vi "Update.vi"(8 "error in (no error)":errorcluster, 10 "Message in":refnum<class "UpdateMessage.lvclass">, 11 "Retiga in":refnum<class "Retiga.lvclass">) -> (0 "error out":errorcluster, 3 "Retiga out":refnum<class "Retiga.lvclass">)   [LabVIEW 2012, in "Retiga.lvclass"]
doc: "The update method processes the command 'update'. \n\nThe command 'update' is used for receiving new values to be set to the private data of the class. This could be seen as a public set method for setting new parameters to the private class data."
uses:
  Retiga.lvclass
  <vilib>/Distrio/Murmex/UpdateMessage/UpdateMessage.lvclass
  Retiga.lvclass/Retiga.ctl
  <vilib>/Distrio/Murmex/Murmex/Murmex.lvclass
panel:
  # "This method is called when the UPDATE\ntrigger is sent. \n\nOverride this method when your component needs to\nrespond to this trigger. \n\nCall parent for proper implementation"
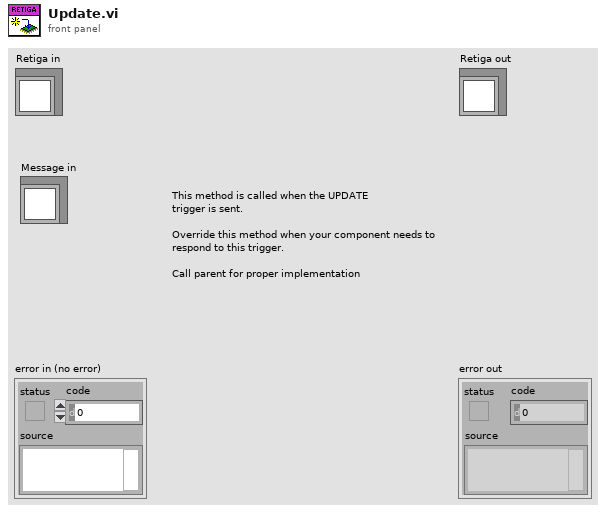
[diagram p1: front panel]
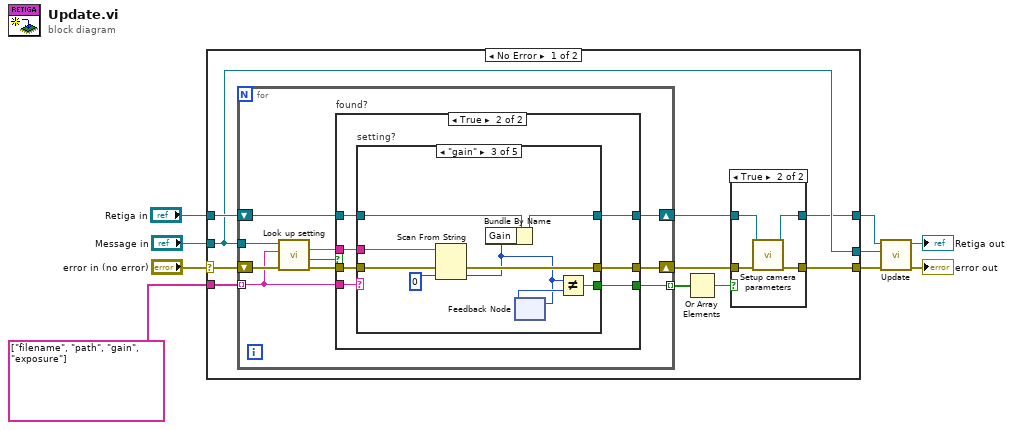
[diagram p0: block diagram]
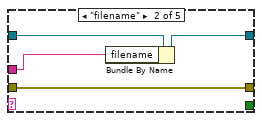
[diagram p5: hidden frame]
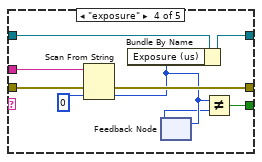
[diagram p6: hidden frame]
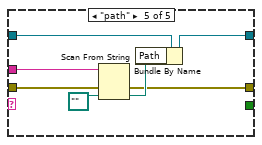
[diagram p7: hidden frame]
diagram:
  n1 = case shown="No Error" "error in (no error)" {
    selector: "error in (no error)" -> [w19 w78]
    tunnel: [w12 w78] -> w6
    tunnel: [w17 w77] -> w5
    tunnel: "Message in" -> [w17 w77]
    tunnel: [w14 w76] -> w3
    tunnel: "Retiga in" -> [w18 w76]
    tunnel: string[] ["filename", "path", "gain", "exposure"] ("key chains") -> [w16 _]
    frame No Error {
      n2 = for {
        tunnel: w17 -> [w34]
        shift-right: [w31] -> w13
        shift-left: w19 -> [w35]
        shift-right: [w30] -> w15
        shift-left: w18 -> [w29]
        tunnel: w16 -> [w28] mode=indexing
        tunnel: [w26] -> w11 mode=indexing
        n3 = call <vilib>:"Look up setting.vi"("error in (no error)"=w35, "tag name"=w28, "UpdateMessage in"=w34) -> ("error out"=w32:errorcluster, "found?"=w33:bool, "value"=w27:string)  [unwired: 5 in, 1 out]
        n4 = case "found?" shown="True" w33 {
          tunnel: w32 -> [w37 w39]
          tunnel: [w37 w40] -> w31
          tunnel: [w36 w42] -> w30
          tunnel: w29 -> [w36 w43]
          tunnel: w28 -> [_ w44]
          tunnel: w27 -> [_ w41]
          tunnel: [_ w38] -> w26
          frame False {
          }
          frame True {
            n5 = case "setting?" shown="\"gain\"" w44 {
              tunnel: w43 -> [w46 w50 w59 w66 w73]
              tunnel: [w46 w49 w58 w64 w69] -> w42
              tunnel: w41 -> [_ w48 w57 w67 w74]
              tunnel: [w45 w47 w54 w63 w70] -> w40
              tunnel: w39 -> [w45 w47 w55 w65 w75]
              tunnel: [_ _ w51 w60 _] -> w38
              frame Default {
              }
              frame "filename" {
                n6 = Bundle By Name(cluster=w50, "filename"=w48) -> (w49:refnum<class "Retiga.lvclass">)
              }
              frame "gain" {
                n7 = Scan From String(input string=w57, error in=w55, default 1=0 ("settings.Gain")) -> (error out=w54:errorcluster, output 1=w52:i32)  [unwired: 2 in, 2 out]
                n8 = Bundle By Name(cluster=w59, "Gain"=w52) -> (w58:refnum<class "Retiga.lvclass">)
                n9 = feedback #1() -> (w53:i32)  [unwired: 1 in]
                n10 = feedback-in #1(w52) -> ()
                n11 = Not Equal?(x=w52, y=w53) -> (x != y?=w51:bool)
              }
              frame "exposure" {
                n12 = Scan From String(input string=w67, error in=w65, default 1=0 ("settings.Gain")) -> (error out=w63:errorcluster, output 1=w62:i32)  [unwired: 2 in, 2 out]
                n13 = Bundle By Name(cluster=w66, "Exposure (us)"=w62) -> (w64:refnum<class "Retiga.lvclass">)
                n14 = feedback-in #2(w62) -> ()
                n15 = feedback #2() -> (w61:i32)  [unwired: 1 in]
                n16 = Not Equal?(x=w62, y=w61) -> (x != y?=w60:bool)
              }
              frame "path" {
                n17 = Scan From String(input string=w74, error in=w75, default 1=path "" ("settings.Path")) -> (error out=w70:errorcluster, output 1=w71:path)  [unwired: 2 in, 2 out]
                n18 = Bundle By Name(cluster=w73, "Path"=w71) -> (w69:refnum<class "Retiga.lvclass">)
              }
            }
          }
        }
      }
      n19 = Or Array Elements(Boolean array=w11) -> (logical OR=w10:bool)
      n20 = case shown="True" w10 {
        tunnel: w15 -> [w21 w25]
        tunnel: [w21 w24] -> w14
        tunnel: w13 -> [w20 w23]
        tunnel: [w20 w22] -> w12
        frame False {
        }
        frame True {
          n21 = call-dynamic "Setup camera parameters.vi"("error in (no error)"=w23, "Retiga in"=w25) -> ("error out"=w22:errorcluster, "Retiga out"=w24:refnum<class "Retiga.lvclass">)  [unwired: 8 in]
        }
      }
    }
    frame Error {
    }
  }
  n22 = call-parent "Update.vi"("error in (no error)"=w6, "Message in"=w5, "Murmex in"=w3) -> ("error out"=→"error out":errorcluster, "Murmex out"=→"Retiga out":refnum<class "Retiga.lvclass">)  [unwired: 7 in]
